vi "initialize CO2 fastClock task.vi"(8 "error in (no error)":errorcluster, 11 "NI in":refnum<class "NI.lvclass">) -> (0 "error out":errorcluster, 3 "NI out":refnum<class "NI.lvclass">)   [LabVIEW 2021, in "NI.lvlib" / "NI.lvclass"]
uses:
  NI.lvclass
  NI.lvclass/NI.ctl
  <vilib>/DAQmx/create/channels.llb/DAQmx Create Channel (CO-Pulse Generation-Frequency).vi
  <vilib>/DAQmx/configure/timing.llb/DAQmx Timing (Implicit).vi
  <vilib>/DAQmx/configure/trigger.llb/DAQmx Start Trigger (Digital Edge).vi
  <resource>/objmgr/daqmx.rc
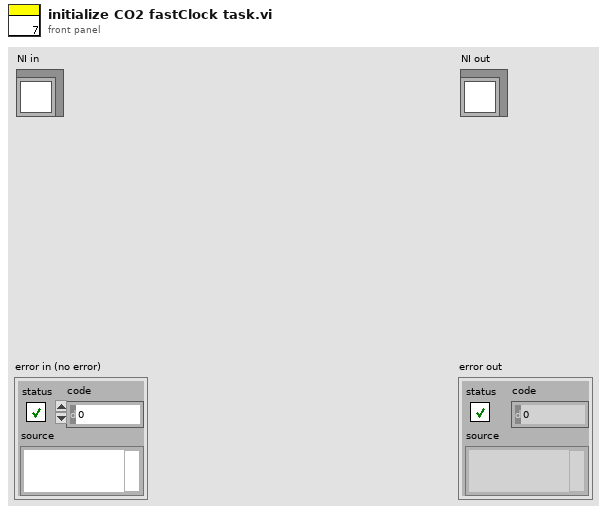
[diagram p1: front panel]
types:
  T1 = typedef "NI.lvlib/NI.lvclass/NI task parameters.ctl" = cluster{"exposure time":dbl, "camera H":dbl, "y line #":dbl, "flyback line #":dbl, "y pixel size":dbl, "z scan #":dbl, "z step size":dbl, "z offset":dbl, "laser all on?":bool, "laser option":bool[]}
  T2 = typedef "NI.lvlib/NI.lvclass/Channel Connection.ctl" = cluster{"Physical Channel":tag, "Terminal":tag, "StartTrigger":tag, "ClockSource":tag}
  T3 = cluster{"fast clock params":cluster{"fast clock rate":dbl, "off time after trigger":dbl, "cam line read time":dbl, "protect ticks #":dbl}, "AO1 laser Connection":T2, "AO2 zy Connection":T2, "AO3 z Connection (deprecated)":T2, "CO1 mainTrig Connection":T2, "CO2 fastClock Connection":T2, "AI phase Connection":T2}
  T4 = cluster{"fast clock rate":dbl, "off time after trigger":dbl, "cam line read time":dbl, "protect ticks #":dbl}
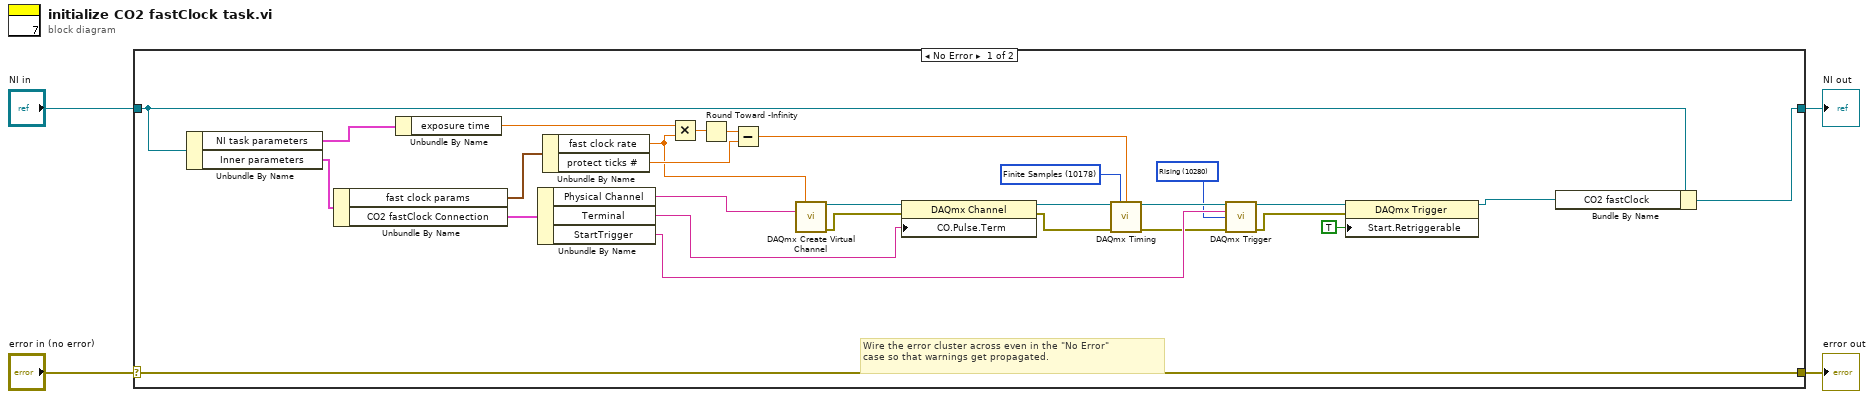
[diagram p0: block diagram]
diagram:
  n1 = case shown="No Error" "error in (no error)" {
    selector: "error in (no error)" -> [w32 w34]
    tunnel: [w32 w34] -> w3
    tunnel: [w20 w33] -> w1
    tunnel: "NI in" -> [w21 w33]
    frame No Error {
      w15 = 10280 items=["Rising"=10280, "Falling"=10171] ("edge")
      w29 = 10178 items=["Finite Samples"=10178, "Continuous Samples"=10123, "Hardware Timed Single Point"=12522] ("sample mode")
      # "Wire the error cluster across even in the \"No Error\"\ncase so that warnings get propagated."
      n2 = Unbundle By Name(w21) -> ("NI task parameters"=w28:T1, "Inner parameters"=w27:T3)
      n3 = Unbundle By Name(w27) -> ("fast clock params"=w12:T4, "CO2 fastClock Connection"=w26:T2)
      n4 = Unbundle By Name(w28) -> ("exposure time"=w11:dbl)
      n5 = Unbundle By Name(w26) -> ("Physical Channel"=w25:tag, "Terminal"=w24:tag, "StartTrigger"=w16:tag)
      n6 = Unbundle By Name(w12) -> ("fast clock rate"=w6:dbl, "protect ticks #"=w8:dbl)
      n7 = Multiply(x=w11, y=w6) -> (x*y=w10:dbl)
      n8 = Round Toward -Infinity(1:w10) -> (0:w9:dbl)
      n9 = Subtract(x=w9, y=w8) -> (x-y=w7:dbl)
      n10 = call-poly <vilib>:"DAQmx Create Virtual Channel.vi"("frequency"=w6, "counter"=w25) -> ("task out"=w31:refnum<k21>, "error out"=w23:errorcluster)  [unwired: 12 in]
      n11 = property class="DAQmx Channel"(reference=w31, error in=w23, "CO.Pulse.Term"=w24) -> (reference out=w30:refnum<k21>, error out=w22:errorcluster)
      n12 = call-poly <vilib>:"DAQmx Timing.vi"("task/channels in"=w30, "sample mode"=w29, "samples per channel"=w7, "error in"=w22) -> ("task out"=w19:refnum<k21>, "error out"=w14:errorcluster)  [unwired: 10 in]
      n13 = call-poly <vilib>:"DAQmx Trigger.vi"("task/channels in"=w19, "source"=w16, "edge"=w15, "error in"=w14) -> ("task out"=w18:refnum<k21>, "error out"=w13:errorcluster)  [unwired: 10 in]
      n14 = property class="DAQmx Trigger"(reference=w18, error in=w13, "Start.Retriggerable"=TRUE) -> (reference out=w5:refnum<k21>)  [unwired: 1 out]
      n15 = Bundle By Name(cluster=w21, "CO2 fastClock"=w5) -> (w20:refnum<class "NI.lvclass">)
    }
    frame Error {
    }
  }
  "error out" <- w3
  "NI out" <- w1
